vi "Memory.Pointer.U64.Read.vi"(8 "error in (no error)":errorcluster, 10 "value":u64, 11 "const U64 Pointer":refnum<class "Memory.Pointer.U64.lvclass">) -> (0 "error out":errorcluster, 2 "value":u64, 3 "U64 Pointer":refnum<class "Memory.Pointer.U64.lvclass">)   [LabVIEW 2016, in "Memory Manager.lvlib" / "Memory.Pointer.U64.lvclass"]
uses:
  Memory.Pointer.U64.lvclass
  C:/Users/Ryan/Documents/Git/Sourcetree/LabVIEW-Memory-Manager/Source/Library/Classes/Pointer/Pointer.Void/Memory.Pointer.Void.lvclass
  Pointer.Void/Memory.Pointer.Void.lvclass/Memory.Pointer.Void.ctl
  Pointer.Void/Memory.Pointer.Void.lvclass
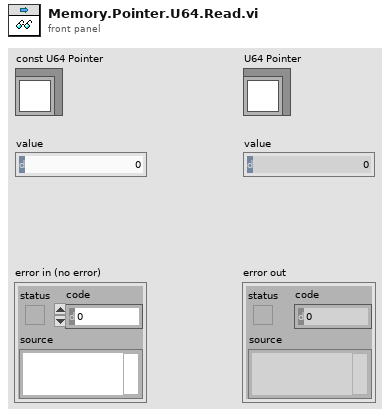
[diagram p1: front panel]
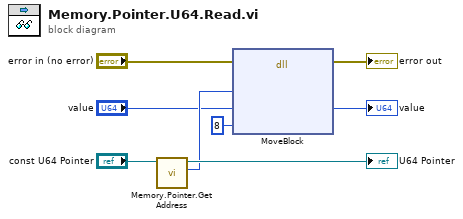
[diagram p0: block diagram]
diagram:
  n1 = call "Memory.Pointer.Get Address.vi"("Pointer in"="const U64 Pointer") -> ("address"=w2:u64, "Pointer out"=→"U64 Pointer":refnum<class "Memory.Pointer.U64.lvclass">)  [unwired: 8 in, 1 out]
  n2 = dll-call lib="LabVIEW" fn="MoveBlock"(error in="error in (no error)", "src"=w2, "dst"="value", "size"=u64 8) -> (error out=→"error out":errorcluster, "dst"=→"value":u64)  [unwired: 5 in, 1 out]
